vi "例3.6 组合框(简易计算器)4.vi"() -> ()   [LabVIEW 2017]
panel:
  in  "功能选择":string(combo)
  out "Result":dbl
  in  "B":dbl
  in  "A":dbl
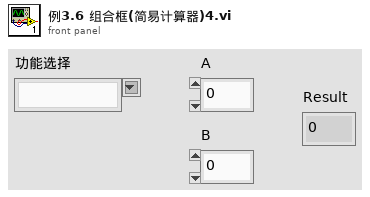
[diagram p1: front panel]
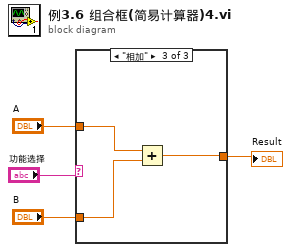
[diagram p0: block diagram]
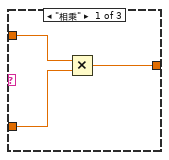
[diagram p2: hidden frame]
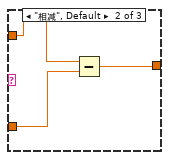
[diagram p3: hidden frame]
diagram:
  n1 = case shown="\"相加\"" "功能选择" {
    tunnel: "A" -> [w7 w10 w13]
    tunnel: "B" -> [w6 w9 w12]
    tunnel: [w5 w8 w11] -> w1
    frame "相乘" {
      n2 = Multiply(x=w7, y=w6) -> (x*y=w5:dbl)
    }
    frame "相减", Default {
      n3 = Subtract(x=w10, y=w9) -> (x-y=w8:dbl)
    }
    frame "相加" {
      n4 = Add(x=w13, y=w12) -> (x+y=w11:dbl)
    }
  }
  "Result" <- w1
